vi "LockIn_#1_data.vi"(1 "Choose Lock-In #3":u16(ring) items=["SR830", "PE7265", "LIA7230", "zurichInst"]) -> (0 "String":string)   [LabVIEW 2019]
uses:
  Instrument_Setup.vi
  Global Variables/Data_Display_global.vi
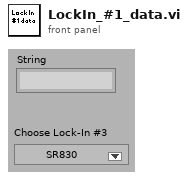
[diagram p1: front panel]
types:
  T1 = typedef "SR830-Settings-Cluster.ctl" = cluster{"VISA":refnum<visa-resource-name>, "Display Channel 2":cluster{" display":i32, " ratio":u16, "output":u16}, "Display Channel 1":cluster{" display":i32, " ratio":u16, "output":u16}, "Time constant":cluster{"time constant\n(10 µs : 0) ":i32, "slope (6 dB/oct)":i32}, "Sensitivity":cluster{"sensitivity\n2nV/fA":i32, "dyn reserve\n(low noise:2)":i16, "ref. phase":ext, "automeasure":bool}, "Offset - Expand.":cluster{"Expand (0: x1)":u16, "Offset/Expand Parameter (1: X)":u16, "Manual Offset (0)":dbl}, "Reference":cluster{"ref. source":bool, "osc.harm# ":u16, "osc. freq":ext, "osc. ampl.":ext, "ref. trigger":u16}, "Lock In 1 sync":cluster{"sync filter":bool, "line filter\n(off:0)":i32}, "Lock In 1 input":cluster{"input":u16, "ground":bool, "couple":bool}}
  T2 = typedef "SR830-Cluster.ctl" = cluster{"Lockin 1":dbl[][], "X1-Display":dbl, "Y1-Display":dbl, "X1 Percent":dbl, "X1 Overload":bool, "Y1 Overload":bool, "Unit X1":string, "Unit X2":string, "Unit X2a":string, "Unit X1a":string, "Sensitivity Setpoint":i16, "X1 Percent 2":dbl, "Y1":dbl, "X1":dbl, "Preamp OVL":bool}
  T3 = typedef "PE7265-Cluster.ctl" = cluster{"Lockin 1":dbl[][], "X1-Display":dbl, "X1 Percent":dbl, "Y1-Display":dbl, "X1 Percent 2":dbl, "Unit X1":string, "Unit X1a":string, "Unit X2":string, "Unit X2a":string, "X1 Overload":bool, "Y1 Overload":bool, "Sensitivity Setpoint":i16, "X1":dbl, "Y1":dbl}
  T4 = cluster{"PE7265 AutoSens at ech step":bool, "PE7265 Sens":i32, "Coupling":bool, "AC Gain":u16, "Auto AC Gain":bool, "Input Device (Voltage Mode)":bool, "Line Frequency":bool, "Input Connector Shells":bool, "PE7265 Input Mode":u16, "Line Frequency\nRejection Filter":u8, "Port":u16, "7265 GPIB Address":i8, "Interface":bool, "Exit":bool, "GPIB Parameter 7260":cluster{"address":string, "delay time":dbl, "mode":i32}, "PE7265 delay after AS":dbl, "VISA session PE7265":refnum<visa-resource-name>, "Slope":u8, "Synchronous TC":bool, "Time Constant":u16, "Reference I/P":u8, "Reference\nHarmonic":u16, "Oscillator Amplitude (Volts rms)":dbl, "Oscillator Frequency (Hz)":dbl, "Ref Unlocked":bool, "Virtual Reference\nMode":bool}
  T5 = typedef "LIA7230-cluster.ctl" = cluster{"Lockin 1":dbl[][], "X1-Display":dbl, "X1 Percent":dbl, "Y1-Display":dbl, "X1 Percent 2":dbl, "Unit X1":string, "Unit X2":string, "X1 Overload":bool, "Y1 Overload":bool, "Sensitivity Setpoint":i16, "X1":dbl, "Y1":dbl, "Channel 3":dbl, "Channel 4":dbl, "Channel 4 Percent":dbl, "Channel 3 Percent ":dbl, "Unit Channel 3":string, "Unit Channel 4":string, "Overload channel 3":bool, "Overload channel 4":bool, "Offsets (ON)":bool, "Sensitivity Setpoint 2":i16}
  T6 = cluster{"Interface":u16, "Port":u16, "Serial Number":string, "IP Address":string, "Line Frequency\nRejection Filter":u8, "Input Mode":u16, "Input Conn. Shells":bool, "Line Frequency":bool, "Auto AC Gain":bool, "AC Gain":u16, "Input Device":bool, "Range":u8, " Auto Sensitivity ":bool, "Auto Measure":bool, "Range 2":u8, " Auto Sensitivity  2":bool, "Slope":u8, "Synchronous TC":bool, "Time Constant":u16, "Slope 2":u8, "Time Constant 2":u16, "Oscillator Amp (V rms)":dbl, "Oscillator Freq (Hz)":dbl, "Reference I/P":u8, "Ref Harm 1":u16, "Ref Harm2":u16, "Virtual Ref.\nMode":bool, "Dual Harmonic/Reference Mode":bool, "Reference Mode":bool, "TRIG OUT\n= Ref Mon":bool, " Auto Phase ":bool, "Reference Phase 1":dbl, "+90 degrees 1":bool, " Auto Phase 2 ":bool, "Reference 2 Phase":dbl, "+90 degrees2":bool, "Auxiliary I/O":bool, "Configuration":bool, "Curve Buffer":bool, "Offsets":bool, "X Channel Offset (%)":sgl, "X Channel Offset":bool, "Y Channel Offset (%)":dbl, "Y Channel Offset":bool, " Auto Offset":bool, "X Channel Offset (%) 2":sgl, "X Channel Offset 2":bool, "Y Channel Offset (%) 2":dbl, "Y Channel Offset 2":bool, " Auto Offset 2":bool, "Display Type channel 1":u16, "Display Type channel 2":u16, "Display Type channel 3":u16, "Display Type channel 4":u16, "Osc Sweeps":bool, "Define Equation1":bool, "Coupling":bool}
  T7 = typedef "Control 3.ctl" = cluster{"Adress":string, "Load Settings from File":bool, "Output_Demod1":enum16{"Aux 1", "Aux 2", "Aux 3", "Aux 4"}, "Input_Demod1":enum16{"Sig In 1", "Curr In 1", "Trigger 1", "Trigger 2", "Aux Out 1", "Aux Out 2", "Aux Out 3", "Aux Out 4", "Aux In 1", "Aux In 2", "Constant"}, "Input_Mode_Demod1":enum16{"single ended", "differential"}, "Bandwith_Mode_Demod1":enum16{"TC", "BW NEP", "BW 3dB"}, "Bandw_Value_demod1":dbl, "Demod1_Range":dbl, "Demod1_Harmonic":dbl, "Trigger_Demod1":enum16{"Manual", "External"}, "osc1_freq":dbl, "osc1_amp":dbl, "Demod1_scaling":dbl, "osc2_freq":dbl, "osc2_amp":dbl, "osc3_freq":dbl, "osc3_amp":dbl, "osc4_freq":dbl, "osc4_amp":dbl, "Demod1_Phase (deg)":dbl, "Demod1_order":ext, "Demod1_coupling":enum16{"DC", "AC"}, "Demod1_shields":enum16{"Ground", "Float"}, "Demod1_input_resistance":enum16{"10M", "50"}, "Demod1_Ref_oscillator":ext, "Demod1_output_imp":enum16{"Disable", "Enable"}, "Demod1_output_diff":enum16{"Disable", "Enable"}, "Demod1_rate":dbl, "Demod1_Output_range":dbl, "Output_Demod2":enum16{"Aux 1", "Aux 2", "Aux 3", "Aux 4"}, "Demod2_input":enum16{"Sig In 1", "Curr In 1", "Trigger 1", "Trigger 2", "Aux Out 1", "Aux Out 2", "Aux Out 3", "Aux Out 4", "Aux In 1", "Aux In 2", "Constant"}, "Input_Mode_Demod2":enum16{"single ended", "differential"}, "Bandwith_Mode_Demod2":enum16{"TC", "BW NEP", "BW 3dB"}, "Bandw_Value_demod2":dbl, "Demod2_Range":dbl, "Demod2_Harmonic":dbl, "Trigger_Demod2":enum16{"Manual", "External"}, "Demod2_scaling":dbl, "Demod2_Phase (deg)":dbl, "Demod2_order":ext, "Demod2_coupling":enum16{"DC", "AC"}, "Demod2_shields":enum16{"Ground", "Float"}, "Demod2_input_resistance":enum16{"10M", "50"}, "Demod2_Ref_oscillator":ext, "Demod2_output_imp":enum16{"Disable", "Enable"}, "Demod2_output_diff":enum16{"Disable", "Enable"}, "Demod2_rate":dbl, "Demod2_Output_range":dbl, "Output_Demod3":enum16{"Aux 1", "Aux 2", "Aux 3", "Aux 4"}, "Demod3_input":enum16{"Sig In 1", "Curr In 1", "Trigger 1", "Trigger 2", "Aux Out 1", "Aux Out 2", "Aux Out 3", "Aux Out 4", "Aux In 1", "Aux In 2", "Constant"}, "Input_Mode_Demod3":enum16{"single ended", "differential"}, "Bandwith_Mode_Demod2":enum16{"TC", "BW NEP", "BW 3dB"}, "Bandw_Value_demod3":dbl, "Demod3_Range":dbl, "Demod3_Harmonic":dbl, "Trigger_Demod3":enum16{"Manual", "External"}, "Demod3_scaling":dbl, "Demod3_Phase (deg)":dbl, "Demod3_order":ext, "Demod3_coupling":enum16{"DC", "AC"}, "Demod3_shields":enum16{"Ground", "Float"}, "Demod3_input_resistance":enum16{"10M", "50"}, "Demod3_Ref_oscillator":ext, "Demod3_output_imp":enum16{"Disable", "Enable"}, "Demod3_output_diff":enum16{"Disable", "Enable"}, "Demod3_rate":dbl, "Demod3_Output_range":dbl, "Output_Demod4":enum16{"Aux 1", "Aux 2", "Aux 3", "Aux 4"}, "Demod4_input":enum16{"Sig In 1", "Curr In 1", "Trigger 1", "Trigger 2", "Aux Out 1", "Aux Out 2", "Aux Out 3", "Aux Out 4", "Aux In 1", "Aux In 2", "Constant"}, "Input_Mode_Demod4":enum16{"single ended", "differential"}, "Bandwith_Mode_Demod4":enum16{"TC", "BW NEP", "BW 3dB"}, "Bandw_Value_demod4":dbl, "Demod4_Range":dbl, "Demod4_Harmonic":dbl, "Trigger_Demod4":enum16{"Manual", "External"}, "Demod4_scaling":dbl, "Demod4_Phase (deg)":dbl, "Demod4_order":ext, "Demod4_coupling":enum16{"DC", "AC"}, "Demod4_shields":enum16{"Ground", "Float"}, "Demod4_input_resistance":enum16{"10M", "50"}, "Demod4_Ref_oscillator":ext, "Demod4_output_imp":enum16{"Disable", "Enable"}, "Demod4_output_diff":enum16{"Disable", "Enable"}, "Demod4_rate":dbl, "Demod4_Output_range":dbl, "Oscillator1_Amp_units":enum16{"Vpk", "Vrms", "VdBm"}, "Oscillator4_Amp_units":enum16{"Vpk", "Vrms", "VdBm"}, "Oscillator2_Amp_units":enum16{"Vpk", "Vrms", "VdBm"}, "Oscillator3_Amp_units":enum16{"Vpk", "Vrms", "VdBm"}, "Demod1_sync_filter":enum16{"Disable", "Enable"}, "Demod 1 (on/off)":bool, "Demod 2 (on/off) ":bool, "Demod 3 (on/off) ":bool, "Demod 4 (on/off) ":bool, " Sigouts 1 (on/off)":bool, " Sigouts 2 (on/off) ":bool, " Sigouts 3 (on/off)":bool, " Sigouts 4 (on/off) ":bool, "Demod2_sync_filter":enum16{"Disable", "Enable"}, "Demod1_auto_outp_rang":enum16{"Disable", "Enable"}, "Demod2_auto_outp_rang ":enum16{"Disable", "Enable"}}
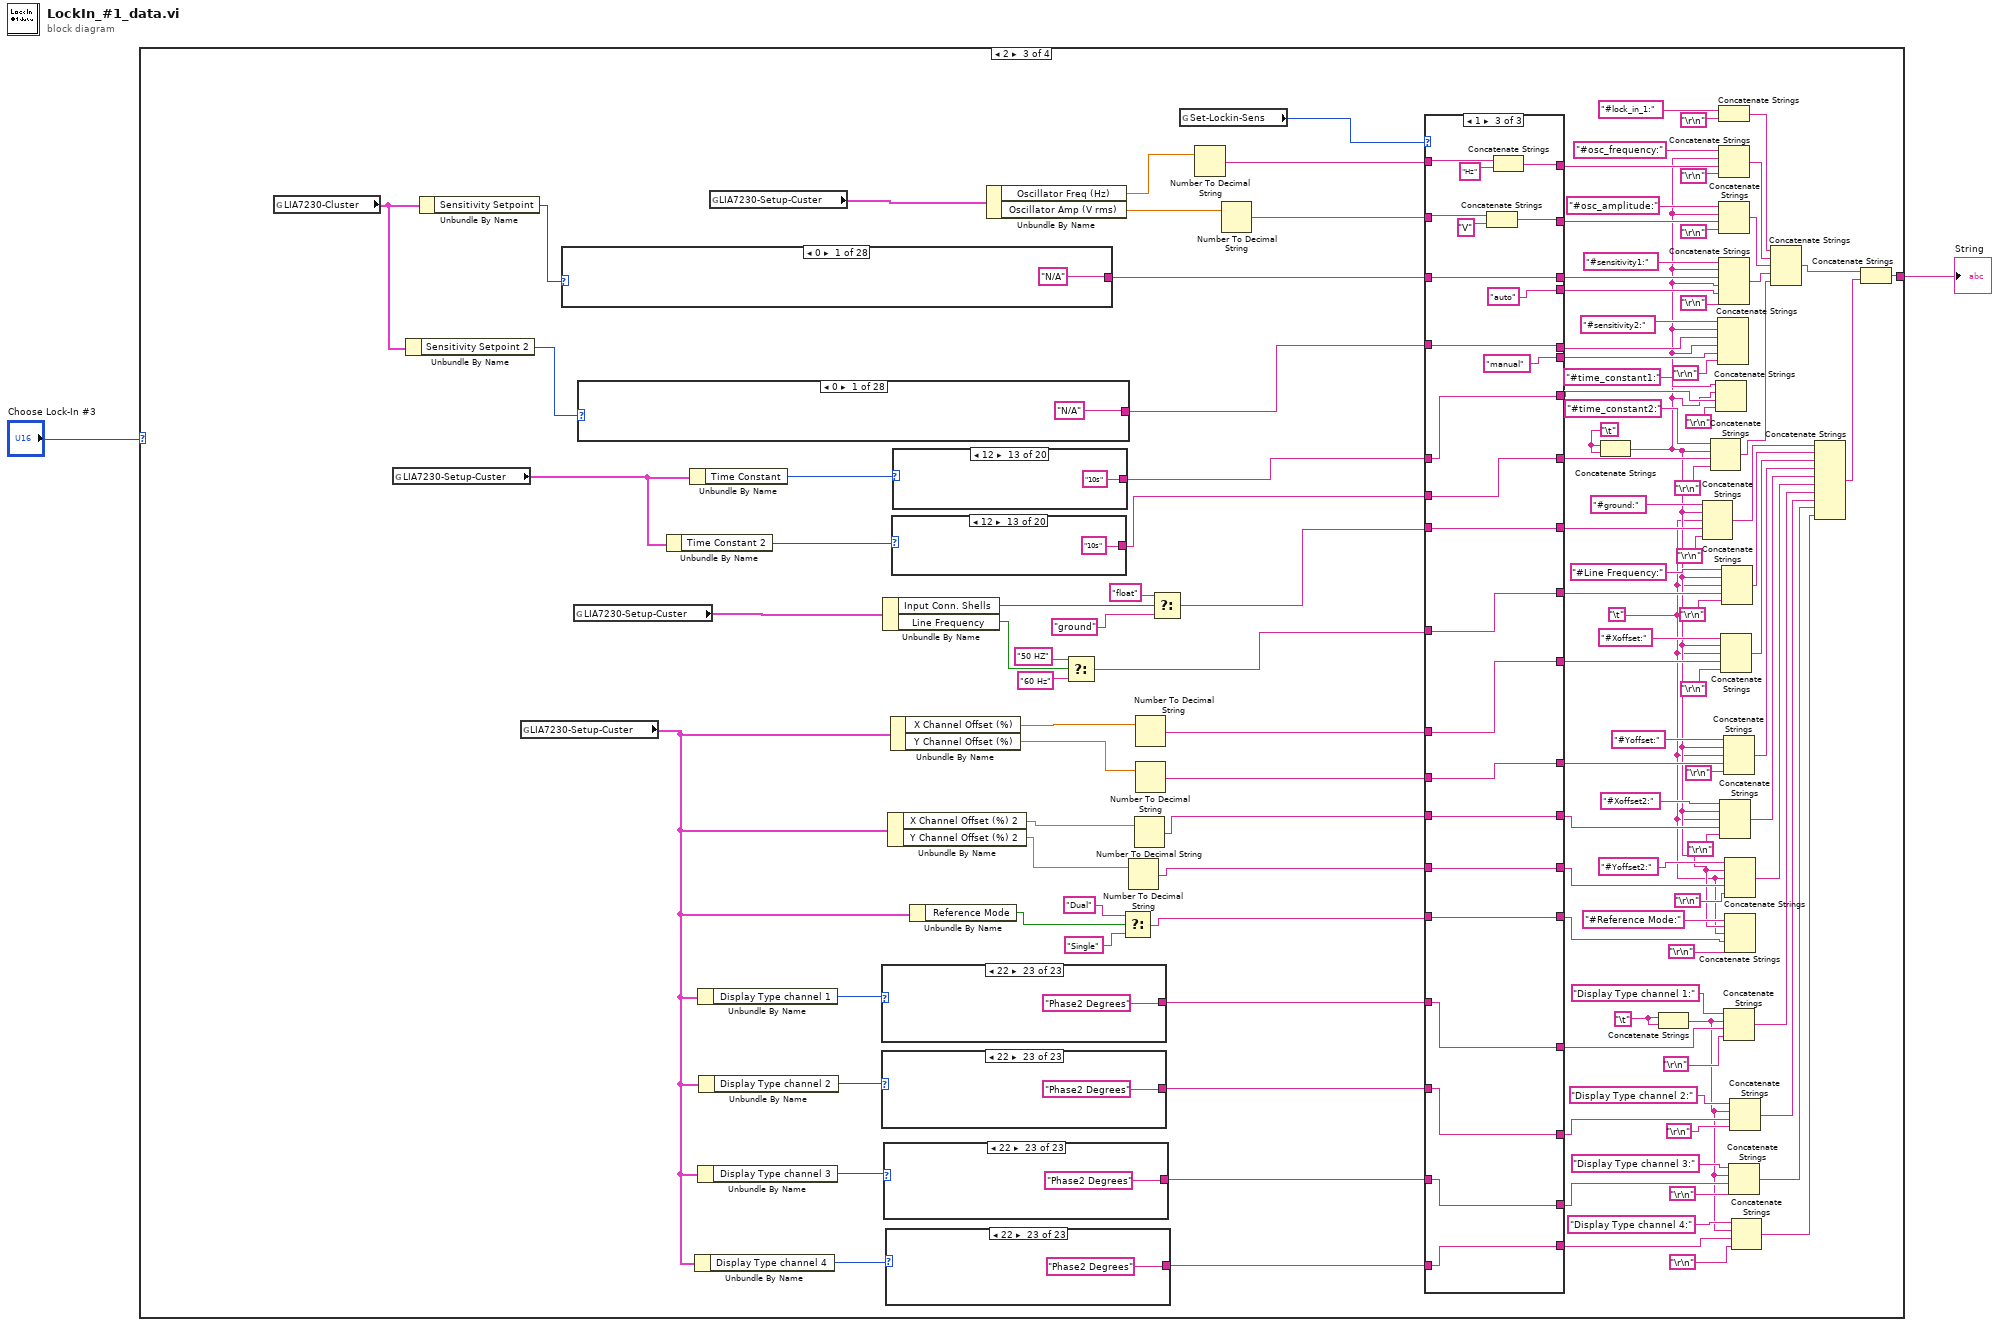
[diagram p0: block diagram]
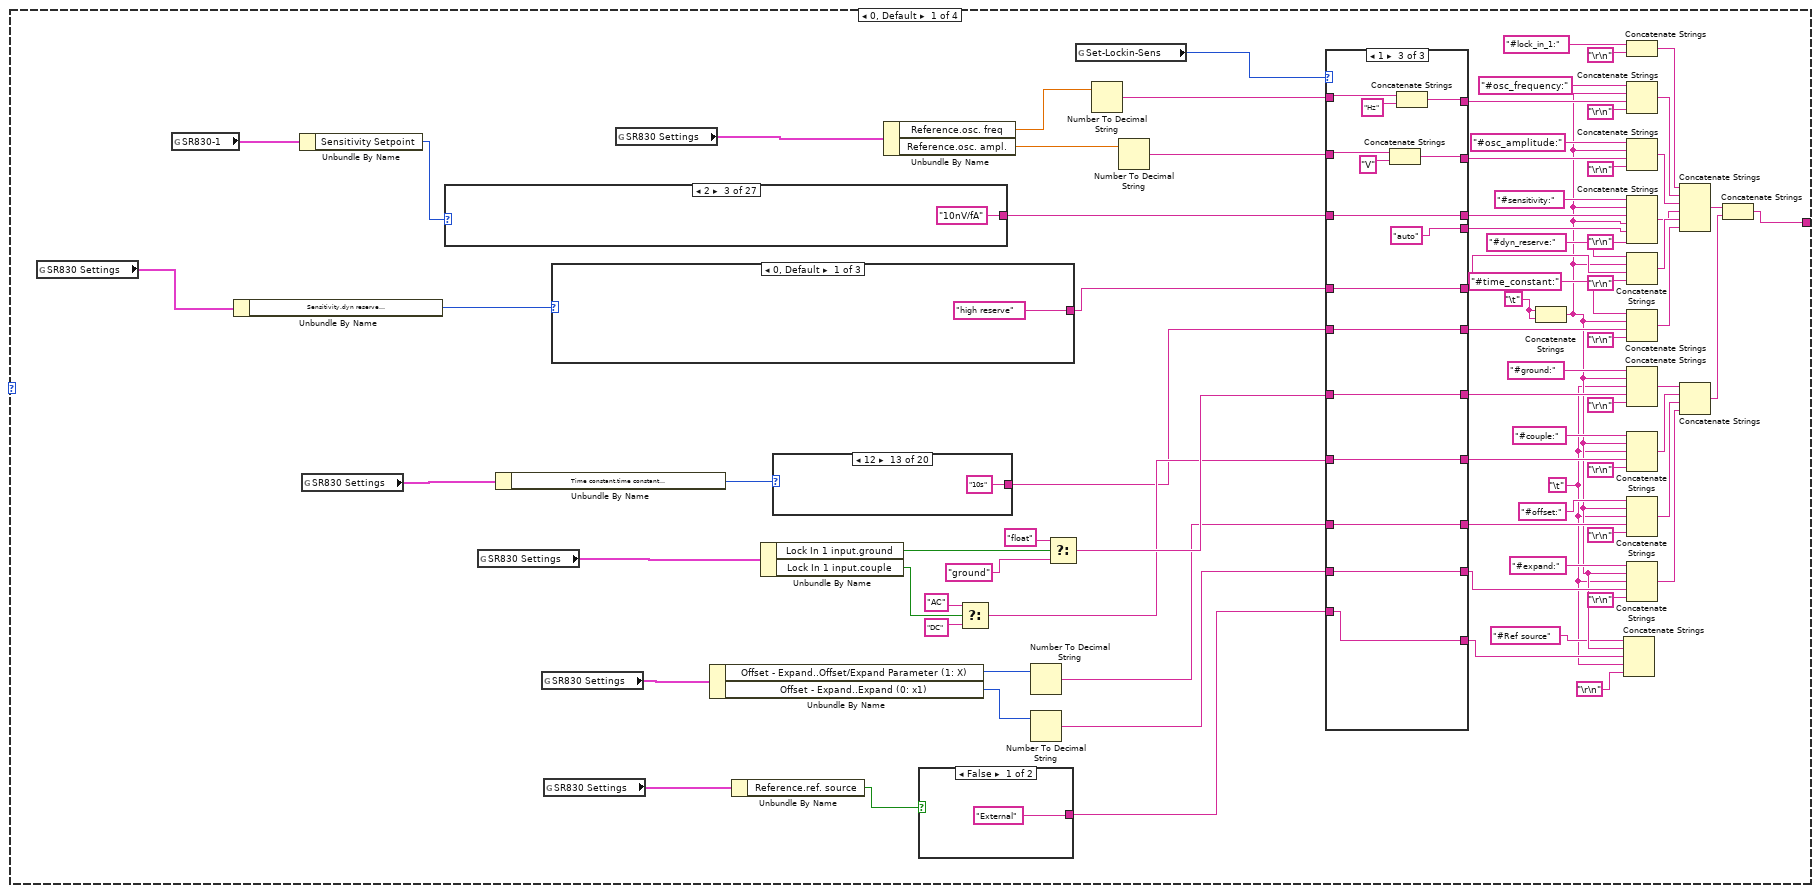
[diagram p2: hidden frame]
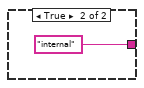
[diagram p3: hidden frame]
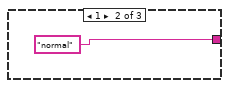
[diagram p4: hidden frame]
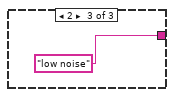
[diagram p5: hidden frame]
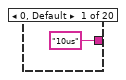
[diagram p6: hidden frame]
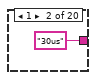
[diagram p7: hidden frame]
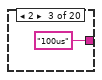
[diagram p8: hidden frame]
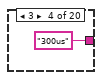
[diagram p9: hidden frame]
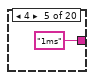
[diagram p10: hidden frame]
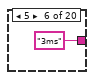
[diagram p11: hidden frame]
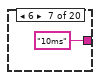
[diagram p12: hidden frame]
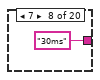
[diagram p13: hidden frame]
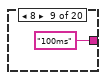
[diagram p14: hidden frame]
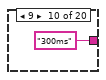
[diagram p15: hidden frame]
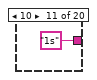
[diagram p16: hidden frame]
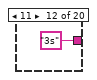
[diagram p17: hidden frame]
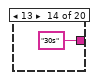
[diagram p18: hidden frame]
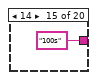
[diagram p19: hidden frame]
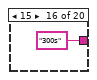
[diagram p20: hidden frame]
diagram:
  n1 = case shown="2" "Choose Lock-In #3" {
    tunnel: [w11 w241 w408 w753] -> w2
    frame 0, Default {
      w3 = "\t"
      w83 = "\t"
      n2 = global read "Instrument_Setup.vi" "SR830 Settings"() -> (w49:T1)
      n3 = global read "Data_Display_global.vi" "SR830-1"() -> (w14:T2)
      n4 = Unbundle By Name(w49) -> ("Sensitivity.dyn reserve\n(low noise:2)"=w16:i16)
      n5 = Unbundle By Name(w14) -> ("Sensitivity Setpoint"=w13:i16)
      n6 = global read "Instrument_Setup.vi" "SR830 Settings"() -> (w55:T1)
      n7 = case shown="2" w13 {
        tunnel: ["2nV/fA" "5nV/fA" "10nV/fA" "20nV/fA" "50nV/fA" "100nV/fA" "200nV/fA" "500nV/fA" "1uV/pA" "2uV/pA" "5uV/pA" "10uV/pA" "20uV/pA" "50uV/pA" "100uV/pA" "200uV/pA" "500uV/pA" "1mV/nA" "2mV/nA" "5mV/nA" "10mV/nA" "20mV/nA" "50mV/nA" "100mV/nA" "200mV/nA" "500mV/nA" "1V/uA"] -> w20
        frame 0, Default {
        }
        frame 1 {
        }
        frame 2 {
        }
        frame 3 {
        }
        frame 4 {
        }
        frame 5 {
        }
        frame 6 {
        }
        frame 7 {
        }
        frame 8 {
        }
        frame 9 {
        }
        frame 10 {
        }
        frame 11 {
        }
        frame 12 {
        }
        frame 13 {
        }
        frame 14 {
        }
        frame 15 {
        }
        frame 16 {
        }
        frame 17 {
        }
        frame 18 {
        }
        frame 19 {
        }
        frame 20 {
        }
        frame 21 {
        }
        frame 22 {
        }
        frame 23 {
        }
        frame 24 {
        }
        frame 25 {
        }
        frame 26 {
        }
      }
      n8 = global read "Instrument_Setup.vi" "SR830 Settings"() -> (w61:T1)
      n9 = Unbundle By Name(w55) -> ("Time constant.time constant\n(10 µs : 0)"=w19:i32)
      n10 = global read "Instrument_Setup.vi" "SR830 Settings"() -> (w68:T1)
      n11 = global read "Instrument_Setup.vi" "SR830 Settings"() -> (w10:T1)
      n12 = case shown="0, Default" w16 {
        tunnel: ["high reserve" "normal" "low noise"] -> w17
        frame 0, Default {
        }
        frame 1 {
        }
        frame 2 {
        }
      }
      n13 = global read "Instrument_Setup.vi" "SR830 Settings"() -> (w47:T1)
      n14 = Unbundle By Name(w68) -> ("Offset - Expand..Offset/Expand Parameter (1: X)"=w40:u16, "Offset - Expand..Expand (0: x1)"=w39:u16)
      n15 = Unbundle By Name(w10) -> ("Reference.ref. source"=w9:bool)
      n16 = Unbundle By Name(w61) -> ("Lock In 1 input.ground"=w62:bool, "Lock In 1 input.couple"=w37:bool)
      n17 = case shown="12" w19 {
        tunnel: ["10us" "30us" "100us" "300us" "1ms" "3ms" "10ms" "30ms" "100ms" "300ms" "1s" "3s" "10s" "30s" "100s" "300s" "1ks" "3ks" "10ks" "30ks"] -> w18
        frame 0, Default {
        }
        frame 1 {
        }
        frame 2 {
        }
        frame 3 {
        }
        frame 4 {
        }
        frame 5 {
        }
        frame 6 {
        }
        frame 7 {
        }
        frame 8 {
        }
        frame 9 {
        }
        frame 10 {
        }
        frame 11 {
        }
        frame 12 {
        }
        frame 13 {
        }
        frame 14 {
        }
        frame 15 {
        }
        frame 16 {
        }
        frame 17 {
        }
        frame 18 {
        }
        frame 19 {
        }
      }
      n18 = Unbundle By Name(w47) -> ("Reference.osc. freq"=w42:ext, "Reference.osc. ampl."=w41:ext)
      n19 = case shown="False" w9 {
        tunnel: ["External" "internal"] -> w8
        frame False {
        }
        frame True {
        }
      }
      n20 = Select(t="AC", s=w37, f="DC") -> (s? t:f=w32:string)
      n21 = Number To Decimal String(number=w40) -> (decimal integer string=w30:string)  [unwired: 1 in]
      n22 = Number To Decimal String(number=w39) -> (decimal integer string=w28:string)  [unwired: 1 in]
      n23 = Select(t="float", s=w62, f="ground") -> (s? t:f=w34:string)
      n24 = global read "Instrument_Setup.vi" "Set-Lockin-Sens"() -> (w36:u16)
      n25 = Number To Decimal String(number=w42) -> (decimal integer string=w26:string)  [unwired: 1 in]
      n26 = Number To Decimal String(number=w41) -> (decimal integer string=w24:string)  [unwired: 1 in]
      n27 = case shown="1" w36 {
        tunnel: w18 -> [w138 w159 w174]
        tunnel: [w138 w159 w174] -> w35
        tunnel: w34 -> [w150 w165 w180]
        tunnel: [w150 w165 w180] -> w33
        tunnel: w32 -> [w149 w164 w179]
        tunnel: [w149 w164 w179] -> w31
        tunnel: [w147 w162 w177] -> w29
        tunnel: w30 -> [w147 w162 w177]
        tunnel: w28 -> [w148 w163 w178]
        tunnel: [w148 w163 w178] -> w27
        tunnel: w26 -> [w145 w155 w170]
        tunnel: [w144 w153 w168] -> w25
        tunnel: w24 -> [w142 w154 w169]
        tunnel: [w141 w152 w167] -> w23
        tunnel: w20 -> [w140 w161 w176]
        tunnel: [w140 w161 w176] -> w22
        tunnel: w17 -> [w139 w160 w175]
        tunnel: [w139 w160 w175] -> w21
        tunnel: ["Command-file" "manual" "auto"] -> w12
        tunnel: w8 -> [w136 w151 w166]
        tunnel: [w136 w151 w166] -> w4
        frame 0, Default {
          n28 = Concatenate Strings(w142, "V" ("String")) -> (w141:string)
          n29 = Concatenate Strings(w145, "Hz" ("String")) -> (w144:string)
        }
        frame 2 {
          n30 = Concatenate Strings(w154, "V" ("String")) -> (w152:string)
          n31 = Concatenate Strings(w155, "Hz" ("String")) -> (w153:string)
        }
        frame 1 {
          n32 = Concatenate Strings(w169, "V" ("String")) -> (w167:string)
          n33 = Concatenate Strings(w170, "Hz" ("String")) -> (w168:string)
        }
      }
      n34 = Concatenate Strings(w83, w83) -> (w6:string)
      n35 = Concatenate Strings("#Ref source", w6, w4, w3, "\r\n") -> ()  [unwired: 1 out]
      n36 = Concatenate Strings("#lock_in_1:", "\r\n") -> (w46:string)
      n37 = Concatenate Strings("#osc_frequency:", w6, w25, "\r\n") -> (w72:string)
      n38 = Concatenate Strings("#osc_amplitude:" ("String"), w6, w23, "\r\n") -> (w73:string)
      n39 = Concatenate Strings("#sensitivity:" ("String"), w6, w22, w6, w12, "\r\n") -> (w74:string)
      n40 = Concatenate Strings("#dyn_reserve:" ("String"), w6, w21, "\r\n") -> (w75:string)
      n41 = Concatenate Strings("#time_constant:" ("String"), w6, w35, "\r\n") -> (w76:string)
      n42 = Concatenate Strings("#ground:" ("String"), w6, w3, w33, "\r\n") -> (w77:string)
      n43 = Concatenate Strings("#couple:" ("String"), w6, w3, w31, "\r\n") -> (w78:string)
      n44 = Concatenate Strings("#offset:" ("String"), w6, w3, w29, "\r\n") -> (w79:string)
      n45 = Concatenate Strings("#expand:" ("String"), w6, w3, w27, "\r\n") -> (w80:string)
      n46 = Concatenate Strings(w46, w72, w73, w74, w75, w76) -> (w81:string)
      n47 = Concatenate Strings(w77, w78, w79, w80) -> (w82:string)
      n48 = Concatenate Strings(w81, w82) -> (w11:string)
    }
    frame 1 {
      w208 = "\t"
      w242 = "\t"
      n49 = global read "Data_Display_global.vi" "PE7265-Cluster"() -> (w187:T3)
      n50 = Unbundle By Name(w187) -> ("Sensitivity Setpoint"=w186:i16)
      n51 = global read "Instrument_Setup.vi" "PE7625-Settings"() -> (w217:T4)
      n52 = case shown="2" w186 {
        tunnel: ["2nV/fA" "5nV/fA" "10nV/fA" "20nV/fA" "50nV/fA" "100nV/fA" "200nV/fA" "500nV/fA" "1uV/pA" "2uV/pA" "5uV/pA" "10uV/pA" "20uV/pA" "50uV/pA" "100uV/pA" "200uV/pA" "500uV/pA" "1mV/nA" "2mV/nA" "5mV/nA" "10mV/nA" "20mV/nA" "50mV/nA" "100mV/nA" "200mV/nA" "500mV/nA" "1V/uA"] -> w191
        frame 0, Default {
        }
        frame 1 {
        }
        frame 2 {
        }
        frame 3 {
        }
        frame 4 {
        }
        frame 5 {
        }
        frame 6 {
        }
        frame 7 {
        }
        frame 8 {
        }
        frame 9 {
        }
        frame 10 {
        }
        frame 11 {
        }
        frame 12 {
        }
        frame 13 {
        }
        frame 14 {
        }
        frame 15 {
        }
        frame 16 {
        }
        frame 17 {
        }
        frame 18 {
        }
        frame 19 {
        }
        frame 20 {
        }
        frame 21 {
        }
        frame 22 {
        }
        frame 23 {
        }
        frame 24 {
        }
        frame 25 {
        }
        frame 26 {
        }
      }
      n53 = global read "Instrument_Setup.vi" "PE7625-Settings"() -> (w223:T4)
      n54 = global read "Instrument_Setup.vi" "PE7625-Settings"() -> (w230:T4)
      n55 = Unbundle By Name(w217) -> ("Time Constant"=w190:u16)
      n56 = global read "Instrument_Setup.vi" "PE7625-Settings"() -> (w212:T4)
      n57 = Unbundle By Name(w230) -> ("AC Gain"=w182:u16)
      n58 = Unbundle By Name(w223) -> ("Input Connector Shells"=w224:bool, "Coupling"=w204:bool)
      n59 = case shown="0, Default" w190 {
        tunnel: ["10us" "20us" "40us" "80us" "160us" "320us" "640us" "5ms" "10ms" "20ms" "50ms" "100ms" "200ms" "500ms" "1s" "2s" "5s" "10s" "20s" "50s" "100s" "200s" "500s" "1ks" "2ks" "5ks" "10ks" "20ks" "50ks" "100ks"] -> w189
        frame 0, Default {
        }
        frame 1 {
        }
        frame 2 {
        }
        frame 3 {
        }
        frame 4 {
        }
        frame 5 {
        }
        frame 6 {
        }
        frame 7 {
        }
        frame 8 {
        }
        frame 9 {
        }
        frame 10 {
        }
        frame 11 {
        }
        frame 12 {
        }
        frame 13 {
        }
        frame 14 {
        }
        frame 15 {
        }
        frame 16 {
        }
        frame 17 {
        }
        frame 18 {
        }
        frame 19 {
        }
        frame 20 {
        }
        frame 21 {
        }
        frame 22 {
        }
        frame 23 {
        }
        frame 24 {
        }
        frame 25 {
        }
        frame 26 {
        }
        frame 27 {
        }
        frame 28 {
        }
        frame 29 {
        }
      }
      n60 = Unbundle By Name(w212) -> ("Oscillator Frequency (Hz)"=w207:dbl, "Oscillator Amplitude (Volts rms)"=w206:dbl)
      n61 = case shown="9" w182 {
        tunnel: ["0dB" "10dB" "20dB" "30dB" "40dB" "50dB" "60dB" "70dB" "80dB" "90dB"] -> w181
        frame 0, Default {
        }
        frame 1 {
        }
        frame 2 {
        }
        frame 3 {
        }
        frame 4 {
        }
        frame 5 {
        }
        frame 6 {
        }
        frame 7 {
        }
        frame 8 {
        }
        frame 9 {
        }
      }
      n62 = Select(t="DC", s=w204, f="AC") -> (s? t:f=w199:string)
      n63 = Select(t="float", s=w224, f="ground") -> (s? t:f=w201:string)
      n64 = global read "Instrument_Setup.vi" "Set-Lockin-Sens"() -> (w203:u16)
      n65 = Number To Decimal String(number=w207) -> (decimal integer string=w196:string)  [unwired: 1 in]
      n66 = Number To Decimal String(number=w206) -> (decimal integer string=w194:string)  [unwired: 1 in]
      n67 = case shown="1" w203 {
        tunnel: w189 -> [w311 w329 w341]
        tunnel: [w311 w329 w341] -> w202
        tunnel: w201 -> [w321 w333 w345]
        tunnel: [w321 w333 w345] -> w200
        tunnel: w199 -> [w320 w332 w344]
        tunnel: [w320 w332 w344] -> w198
        tunnel: [w319 w331 w343] -> w197
        tunnel: w181 -> [w319 w331 w343]
        tunnel: w196 -> [w317 w325 w337]
        tunnel: [w316 w323 w335] -> w195
        tunnel: w194 -> [w314 w324 w336]
        tunnel: [w313 w322 w334] -> w193
        tunnel: w191 -> [w312 w330 w342]
        tunnel: [w312 w330 w342] -> w192
        tunnel: ["Command-file" "manual" "auto"] -> w184
        frame 0, Default {
          n68 = Concatenate Strings(w314, "V" ("String")) -> (w313:string)
          n69 = Concatenate Strings(w317, "Hz" ("String")) -> (w316:string)
        }
        frame 2 {
          n70 = Concatenate Strings(w324, "V" ("String")) -> (w322:string)
          n71 = Concatenate Strings(w325, "Hz" ("String")) -> (w323:string)
        }
        frame 1 {
          n72 = Concatenate Strings(w336, "V" ("String")) -> (w334:string)
          n73 = Concatenate Strings(w337, "Hz" ("String")) -> (w335:string)
        }
      }
      n74 = Concatenate Strings(w242, w242) -> (w185:string)
      n75 = Concatenate Strings("#lock_in_1:", "\r\n") -> (w211:string)
      n76 = Concatenate Strings("#osc_frequency:", w185, w195, "\r\n") -> (w233:string)
      n77 = Concatenate Strings("#osc_amplitude:" ("String"), w185, w193, "\r\n") -> (w234:string)
      n78 = Concatenate Strings("#sensitivity:" ("String"), w185, w192, w185, w184, "\r\n") -> (w235:string)
      n79 = Concatenate Strings("#time_constant:" ("String"), w185, w202, "\r\n") -> (w183:string)
      n80 = Concatenate Strings("#ground:" ("String"), w185, w208, w200, "\r\n") -> (w236:string)
      n81 = Concatenate Strings("#couple:" ("String"), w185, w208, w198, "\r\n") -> (w237:string)
      n82 = Concatenate Strings("#AC Gain" ("String"), w185, w208, w197, "\r\n") -> (w238:string)
      n83 = Concatenate Strings(w211, w233, w234, w235, w183) -> (w239:string)
      n84 = Concatenate Strings(w236, w237, w238) -> (w240:string)
      n85 = Concatenate Strings(w239, w240) -> (w241:string)
    }
    frame 2 {
      w362 = "\t"
      w374 = "\t"
      w469 = "\t"
      n86 = global read "Data_Display_global.vi" "LIA7230-Cluster"() -> (w407:T5)
      n87 = global read "Instrument_Setup.vi" "LIA7230-Setup-Custer"() -> (w399:T6)
      n88 = Unbundle By Name(w407) -> ("Sensitivity Setpoint 2"=w406:i16)
      n89 = Unbundle By Name(w407) -> ("Sensitivity Setpoint"=w410:i16)
      n90 = global read "Instrument_Setup.vi" "LIA7230-Setup-Custer"() -> (w371:T6)
      n91 = case shown="0" w410 {
        tunnel: ["N/A" "2nV/fA" "5nV/fA" "10nV/fA" "20nV/fA" "50nV/fA" "100nV/fA" "200nV/fA" "500nV/fA" "1uV/pA" "2uV/pA" "5uV/pA" "10uV/pA" "20uV/pA" "50uV/pA" "100uV/pA" "200uV/pA" "500uV/pA" "1mV/nA" "2mV/nA" "5mV/nA" "10mV/nA" "20mV/nA" "50mV/nA" "100mV/nA" "200mV/nA" "500mV/nA" "1V/uA"] -> w414
        frame 0 {
        }
        frame 1, Default {
        }
        frame 2 {
        }
        frame 3 {
        }
        frame 4 {
        }
        frame 5 {
        }
        frame 6 {
        }
        frame 7 {
        }
        frame 8 {
        }
        frame 9 {
        }
        frame 10 {
        }
        frame 11 {
        }
        frame 12 {
        }
        frame 13 {
        }
        frame 14 {
        }
        frame 15 {
        }
        frame 16 {
        }
        frame 17 {
        }
        frame 18 {
        }
        frame 19 {
        }
        frame 20 {
        }
        frame 21 {
        }
        frame 22 {
        }
        frame 23 {
        }
        frame 24 {
        }
        frame 25 {
        }
        frame 26 {
        }
        frame 27 {
        }
      }
      n92 = global read "Instrument_Setup.vi" "LIA7230-Setup-Custer"() -> (w450:T6)
      n93 = case shown="0" w406 {
        tunnel: ["N/A" "2nV/fA" "5nV/fA" "10nV/fA" "20nV/fA" "50nV/fA" "100nV/fA" "200nV/fA" "500nV/fA" "1uV/pA" "2uV/pA" "5uV/pA" "10uV/pA" "20uV/pA" "50uV/pA" "100uV/pA" "200uV/pA" "500uV/pA" "1mV/nA" "2mV/nA" "5mV/nA" "10mV/nA" "20mV/nA" "50mV/nA" "100mV/nA" "200mV/nA" "500mV/nA" "1V/uA"] -> w405
        frame 0 {
        }
        frame 1, Default {
        }
        frame 2 {
        }
        frame 3 {
        }
        frame 4 {
        }
        frame 5 {
        }
        frame 6 {
        }
        frame 7 {
        }
        frame 8 {
        }
        frame 9 {
        }
        frame 10 {
        }
        frame 11 {
        }
        frame 12 {
        }
        frame 13 {
        }
        frame 14 {
        }
        frame 15 {
        }
        frame 16 {
        }
        frame 17 {
        }
        frame 18 {
        }
        frame 19 {
        }
        frame 20 {
        }
        frame 21 {
        }
        frame 22 {
        }
        frame 23 {
        }
        frame 24 {
        }
        frame 25 {
        }
        frame 26 {
        }
        frame 27 {
        }
      }
      n94 = Unbundle By Name(w399) -> ("Time Constant 2"=w398:u16)
      n95 = Unbundle By Name(w399) -> ("Time Constant"=w413:u16)
      n96 = Unbundle By Name(w371) -> ("Display Type channel 4"=w368:u16)
      n97 = Unbundle By Name(w371) -> ("Display Type channel 1"=w372:u16)
      n98 = Unbundle By Name(w371) -> ("Display Type channel 3"=w369:u16)
      n99 = Unbundle By Name(w371) -> ("Display Type channel 2"=w370:u16)
      n100 = global read "Instrument_Setup.vi" "LIA7230-Setup-Custer"() -> (w440:T6)
      n101 = case shown="22" w372 {
        tunnel: ["X%" "Y%" "X Calibrated" "Y Calibrated" "Mag %" "Mag Calibrated" "Phase Degree" "Ratio" "Log Ratio" "ADC 1" "ADC 2" "ADC 3" "ADC 4" "Noise %" "Noise Calibrated" "Ref Frequency" "Equation 1" "Equation 2" "X2 %" "Y2 %" "Mag2 %" "Mag2 Calibrated" "Phase2 Degrees"] -> w367
        frame 0, Default {
        }
        frame 1 {
        }
        frame 2 {
        }
        frame 3 {
        }
        frame 4 {
        }
        frame 5 {
        }
        frame 6 {
        }
        frame 7 {
        }
        frame 8 {
        }
        frame 9 {
        }
        frame 10 {
        }
        frame 11 {
        }
        frame 12 {
        }
        frame 13 {
        }
        frame 14 {
        }
        frame 15 {
        }
        frame 16 {
        }
        frame 17 {
        }
        frame 18 {
        }
        frame 19 {
        }
        frame 20 {
        }
        frame 21 {
        }
        frame 22 {
        }
      }
      n102 = case shown="22" w370 {
        tunnel: ["X%" "Y%" "X Calibrated" "Y Calibrated" "Mag %" "Mag Calibrated" "Phase Degree" "Ratio" "Log Ratio" "ADC 1" "ADC 2" "ADC 3" "ADC 4" "Noise %" "Noise Calibrated" "Ref Frequency" "Equation 1" "Equation 2" "X2 %" "Y2 %" "Mag2 %" "Mag2 Calibrated" "Phase2 Degrees"] -> w366
        frame 0, Default {
        }
        frame 1 {
        }
        frame 2 {
        }
        frame 3 {
        }
        frame 4 {
        }
        frame 5 {
        }
        frame 6 {
        }
        frame 7 {
        }
        frame 8 {
        }
        frame 9 {
        }
        frame 10 {
        }
        frame 11 {
        }
        frame 12 {
        }
        frame 13 {
        }
        frame 14 {
        }
        frame 15 {
        }
        frame 16 {
        }
        frame 17 {
        }
        frame 18 {
        }
        frame 19 {
        }
        frame 20 {
        }
        frame 21 {
        }
        frame 22 {
        }
      }
      n103 = Unbundle By Name(w450) -> ("Input Conn. Shells"=w451:bool, "Line Frequency"=w430:bool)
      n104 = case shown="22" w369 {
        tunnel: ["X%" "Y%" "X Calibrated" "Y Calibrated" "Mag %" "Mag Calibrated" "Phase Degree" "Ratio" "Log Ratio" "ADC 1" "ADC 2" "ADC 3" "ADC 4" "Noise %" "Noise Calibrated" "Ref Frequency" "Equation 1" "Equation 2" "X2 %" "Y2 %" "Mag2 %" "Mag2 Calibrated" "Phase2 Degrees"] -> w365
        frame 0, Default {
        }
        frame 1 {
        }
        frame 2 {
        }
        frame 3 {
        }
        frame 4 {
        }
        frame 5 {
        }
        frame 6 {
        }
        frame 7 {
        }
        frame 8 {
        }
        frame 9 {
        }
        frame 10 {
        }
        frame 11 {
        }
        frame 12 {
        }
        frame 13 {
        }
        frame 14 {
        }
        frame 15 {
        }
        frame 16 {
        }
        frame 17 {
        }
        frame 18 {
        }
        frame 19 {
        }
        frame 20 {
        }
        frame 21 {
        }
        frame 22 {
        }
      }
      n105 = case shown="22" w368 {
        tunnel: ["X%" "Y%" "X Calibrated" "Y Calibrated" "Mag %" "Mag Calibrated" "Phase Degree" "Ratio" "Log Ratio" "ADC 1" "ADC 2" "ADC 3" "ADC 4" "Noise %" "Noise Calibrated" "Ref Frequency" "Equation 1" "Equation 2" "X2 %" "Y2 %" "Mag2 %" "Mag2 Calibrated" "Phase2 Degrees"] -> w364
        frame 0, Default {
        }
        frame 1 {
        }
        frame 2 {
        }
        frame 3 {
        }
        frame 4 {
        }
        frame 5 {
        }
        frame 6 {
        }
        frame 7 {
        }
        frame 8 {
        }
        frame 9 {
        }
        frame 10 {
        }
        frame 11 {
        }
        frame 12 {
        }
        frame 13 {
        }
        frame 14 {
        }
        frame 15 {
        }
        frame 16 {
        }
        frame 17 {
        }
        frame 18 {
        }
        frame 19 {
        }
        frame 20 {
        }
        frame 21 {
        }
        frame 22 {
        }
      }
      n106 = Unbundle By Name(w371) -> ("X Channel Offset (%) 2"=w391:sgl, "Y Channel Offset (%) 2"=w387:dbl)
      n107 = Unbundle By Name(w371) -> ("X Channel Offset (%)"=w433:sgl, "Y Channel Offset (%)"=w432:dbl)
      n108 = case shown="12" w398 {
        tunnel: ["10us" "30us" "100us" "300us" "1ms" "3ms" "10ms" "30ms" "100ms" "300ms" "1s" "3s" "10s" "30s" "100s" "300s" "1ks" "3ks" "10ks" "30ks"] -> w397
        frame 0, Default {
        }
        frame 1 {
        }
        frame 2 {
        }
        frame 3 {
        }
        frame 4 {
        }
        frame 5 {
        }
        frame 6 {
        }
        frame 7 {
        }
        frame 8 {
        }
        frame 9 {
        }
        frame 10 {
        }
        frame 11 {
        }
        frame 12 {
        }
        frame 13 {
        }
        frame 14 {
        }
        frame 15 {
        }
        frame 16 {
        }
        frame 17 {
        }
        frame 18 {
        }
        frame 19 {
        }
      }
      n109 = case shown="12" w413 {
        tunnel: ["10us" "30us" "100us" "300us" "1ms" "3ms" "10ms" "30ms" "100ms" "300ms" "1s" "3s" "10s" "30s" "100s" "300s" "1ks" "3ks" "10ks" "30ks"] -> w412
        frame 0, Default {
        }
        frame 1 {
        }
        frame 2 {
        }
        frame 3 {
        }
        frame 4 {
        }
        frame 5 {
        }
        frame 6 {
        }
        frame 7 {
        }
        frame 8 {
        }
        frame 9 {
        }
        frame 10 {
        }
        frame 11 {
        }
        frame 12 {
        }
        frame 13 {
        }
        frame 14 {
        }
        frame 15 {
        }
        frame 16 {
        }
        frame 17 {
        }
        frame 18 {
        }
        frame 19 {
        }
      }
      n110 = Unbundle By Name(w371) -> ("Reference Mode"=w381:bool)
      n111 = Unbundle By Name(w440) -> ("Oscillator Freq (Hz)"=w435:dbl, "Oscillator Amp (V rms)"=w434:dbl)
      n112 = Select(t="50 HZ", s=w430, f="60 Hz") -> (s? t:f=w425:string)
      n113 = Select(t="Dual", s=w381, f="Single") -> (s? t:f=w378:string)
      n114 = Number To Decimal String(number=w387) -> (decimal integer string=w386:string)  [unwired: 1 in]
      n115 = Number To Decimal String(number=w391) -> (decimal integer string=w390:string)  [unwired: 1 in]
      n116 = Number To Decimal String(number=w433) -> (decimal integer string=w423:string)  [unwired: 1 in]
      n117 = Number To Decimal String(number=w432) -> (decimal integer string=w421:string)  [unwired: 1 in]
      n118 = Select(t="float", s=w451, f="ground") -> (s? t:f=w427:string)
      n119 = global read "Instrument_Setup.vi" "Set-Lockin-Sens"() -> (w429:u16)
      n120 = Number To Decimal String(number=w435) -> (decimal integer string=w419:string)  [unwired: 1 in]
      n121 = Number To Decimal String(number=w434) -> (decimal integer string=w417:string)  [unwired: 1 in]
      n122 = case shown="1" w429 {
        tunnel: w412 -> [w666 w689 w712]
        tunnel: [w665 w688 w711] -> w428
        tunnel: w427 -> [w680 w703 w726]
        tunnel: [w680 w703 w726] -> w426
        tunnel: w425 -> [w679 w702 w725]
        tunnel: [w679 w702 w725] -> w424
        tunnel: [w677 w700 w723] -> w422
        tunnel: w423 -> [w677 w700 w723]
        tunnel: w421 -> [w678 w701 w724]
        tunnel: [w678 w701 w724] -> w420
        tunnel: w419 -> [w675 w695 w718]
        tunnel: [w674 w693 w716] -> w418
        tunnel: w417 -> [w672 w694 w717]
        tunnel: [w671 w692 w715] -> w416
        tunnel: w414 -> [w670 w699 w722]
        tunnel: [w670 w699 w722] -> w415
        tunnel: ["Command-file" "manual" "auto"] -> w409
        tunnel: w405 -> [w668 w691 w714]
        tunnel: [w668 w691 w714] -> w402
        tunnel: ["manual" "manual" "manual"] -> w401
        tunnel: w397 -> [w665 w688 w711]
        tunnel: [w666 w689 w712] -> w394
        tunnel: w390 -> [w664 w687 w710]
        tunnel: [w664 w687 w710] -> w389
        tunnel: w386 -> [w663 w686 w709]
        tunnel: [w663 w686 w709] -> w383
        tunnel: w378 -> [w662 w685 w708]
        tunnel: [w662 w685 w708] -> w373
        tunnel: w367 -> [w661 w684 w707]
        tunnel: w366 -> [w660 w683 w706]
        tunnel: w365 -> [w659 w682 w705]
        tunnel: w364 -> [w658 w681 w704]
        tunnel: [w661 w684 w707] -> w361
        tunnel: [w660 w683 w706] -> w358
        tunnel: [w659 w682 w705] -> w355
        tunnel: [w658 w681 w704] -> w351
        frame 0, Default {
          n123 = Concatenate Strings(w672, "V" ("String")) -> (w671:string)
          n124 = Concatenate Strings(w675, "Hz" ("String")) -> (w674:string)
        }
        frame 2 {
          n125 = Concatenate Strings(w694, "V" ("String")) -> (w692:string)
          n126 = Concatenate Strings(w695, "Hz" ("String")) -> (w693:string)
        }
        frame 1 {
          n127 = Concatenate Strings(w717, "V" ("String")) -> (w715:string)
          n128 = Concatenate Strings(w718, "Hz" ("String")) -> (w716:string)
        }
      }
      n129 = Concatenate Strings(w469, w469) -> (w375:string)
      n130 = Concatenate Strings(w362, w362) -> (w352:string)
      n131 = Concatenate Strings("#ground:" ("String"), w375, w374, w426, "\r\n") -> (w463:string)
      n132 = Concatenate Strings("#time_constant2:" ("String"), w375, w428, "\r\n") -> (w400:string)
      n133 = Concatenate Strings("#time_constant1:" ("String"), w375, w394, "\r\n") -> ()  [unwired: 1 out]
      n134 = Concatenate Strings("#sensitivity2:" ("String"), w375, w402, w375, w401, "\r\n") -> ()  [unwired: 1 out]
      n135 = Concatenate Strings("#lock_in_1:", "\r\n") -> (w439:string)
      n136 = Concatenate Strings("#osc_frequency:", w375, w418, "\r\n") -> (w460:string)
      n137 = Concatenate Strings("#osc_amplitude:" ("String"), w375, w416, "\r\n") -> (w461:string)
      n138 = Concatenate Strings("#sensitivity1:" ("String"), w375, w415, w375, w409, "\r\n") -> (w462:string)
      n139 = Concatenate Strings("#Xoffset2:" ("String"), w375, w374, w389, "\r\n") -> (w393:string)
      n140 = Concatenate Strings("#Xoffset:" ("String"), w375, w374, w422, "\r\n") -> (w465:string)
      n141 = Concatenate Strings("#Line Frequency:" ("String"), w375, w374, w424, "\r\n") -> (w464:string)
      n142 = Concatenate Strings("#Yoffset:" ("String"), w375, w374, w420, "\r\n") -> (w466:string)
      n143 = Concatenate Strings("Display Type channel 1:", w352, w361, "\r\n") -> (w349:string)
      n144 = Concatenate Strings("#Yoffset2:" ("String"), w375, w374, w383, "\r\n") -> (w385:string)
      n145 = Concatenate Strings("#Reference Mode:" ("String"), w375, w374, w373, "\r\n") -> ()  [unwired: 1 out]
      n146 = Concatenate Strings("Display Type channel 3:", w352, w355, "\r\n") -> (w347:string)
      n147 = Concatenate Strings("Display Type channel 2:", w352, w358, "\r\n") -> (w348:string)
      n148 = Concatenate Strings("Display Type channel 4:", w352, w351, "\r\n") -> (w346:string)
      n149 = Concatenate Strings(w439, w460, w461, w462, w400) -> (w467:string)
      n150 = Concatenate Strings(w463, w464, w465, w466, w393, w385, w349, w348, w347, w346) -> (w468:string)
      n151 = Concatenate Strings(w467, w468) -> (w408:string)
    }
    frame 3 {
      w763 = "\t"
      w787 = "\t"
      n152 = global read "Instrument_Setup.vi" "zurichInst-1-Settings"() -> (w732:T7)
      n153 = Unbundle By Name(w732) -> ("osc1_freq"=w750:dbl, "osc1_amp"=w748:dbl)
      n154 = Unbundle By Name(w732) -> ("osc2_freq"=w746:dbl, "osc2_amp"=w745:dbl)
      n155 = Unbundle By Name(w732) -> ("Demod1_shields"=w734:enum16{"Ground", "Float"})
      n156 = Unbundle By Name(w732) -> ("Demod1_coupling"=w731:enum16{"DC", "AC"})
      n157 = Number To Decimal String(number=w750) -> (decimal integer string=w749:string)  [unwired: 1 in]
      n158 = Number To Decimal String(number=w748) -> (decimal integer string=w747:string)  [unwired: 1 in]
      n159 = Number To Decimal String(number=w745) -> (decimal integer string=w743:string)  [unwired: 1 in]
      n160 = Number To Decimal String(number=w746) -> (decimal integer string=w744:string)  [unwired: 1 in]
      n161 = case shown="\"Float\"" w734 {
        tunnel: ["Ground" "Float"] -> w733
        frame "Ground", Default {
        }
        frame "Float" {
        }
      }
      n162 = case shown="\"DC\", Default" w731 {
        tunnel: ["DC" "AC"] -> w730
        frame "DC", Default {
        }
        frame "AC" {
        }
      }
      n163 = case shown="2" 1 {
        tunnel: "Not implementet yet" -> [w799 w823 w841]
        tunnel: [w799 w823 w841] -> w762
        tunnel: w733 -> [w809 w827 w845]
        tunnel: [w809 w827 w845] -> w761
        tunnel: w730 -> [w808 w826 w844]
        tunnel: [w808 w826 w844] -> w760
        tunnel: [w807 w825 w843] -> w759
        tunnel: "Not implementet yet" -> [w807 w825 w843]
        tunnel: w749 -> [w805 w819 w837]
        tunnel: [w804 w817 w835] -> w758
        tunnel: w747 -> [w802 w818 w836]
        tunnel: [w801 w816 w834] -> w757
        tunnel: "Nd" -> [w800 w824 w842]
        tunnel: [w800 w824 w842] -> w756
        tunnel: ["Command-file" "manual" "auto"] -> w754
        tunnel: w744 -> [w797 w814 w833]
        tunnel: w743 -> [w796 w813 w831]
        tunnel: [w795 w812 w829] -> w741
        tunnel: [w794 w811 w828] -> w737
        frame 0, Default {
          n164 = Concatenate Strings(w802, "V" ("String")) -> (w801:string)
          n165 = Concatenate Strings(w805, "Hz" ("String")) -> (w804:string)
          n166 = Concatenate Strings(w796, "V" ("String")) -> (w794:string)
          n167 = Concatenate Strings(w797, "Hz" ("String")) -> (w795:string)
        }
        frame 2 {
          n168 = Concatenate Strings(w818, "V" ("String")) -> (w816:string)
          n169 = Concatenate Strings(w813, "V" ("String")) -> (w811:string)
          n170 = Concatenate Strings(w814, "Hz" ("String")) -> (w812:string)
          n171 = Concatenate Strings(w819, "Hz" ("String")) -> (w817:string)
        }
        frame 1 {
          n172 = Concatenate Strings(w837, "Hz" ("String")) -> (w835:string)
          n173 = Concatenate Strings(w831, "V" ("String")) -> (w828:string)
          n174 = Concatenate Strings(w833, "Hz" ("String")) -> (w829:string)
          n175 = Concatenate Strings(w836, "V" ("String")) -> (w834:string)
        }
      }
      n176 = Concatenate Strings(w787, w787) -> (w738:string)
      n177 = Concatenate Strings("#osc2_amplitude:" ("String"), w738, w737, "\r\n") -> ()  [unwired: 1 out]
      n178 = Concatenate Strings("#osc2_frequency:", w738, w741, "\r\n") -> ()  [unwired: 1 out]
      n179 = Concatenate Strings("#time_constant:" ("String"), w738, w762, "\r\n") -> (w727:string)
      n180 = Concatenate Strings("#ground_Demod1:" ("String"), w738, w763, w761, "\r\n") -> (w782:string)
      n181 = Concatenate Strings("#couple_Demod1:" ("String"), w738, w763, w760, "\r\n") -> (w783:string)
      n182 = Concatenate Strings("#AC Gain" ("String"), w738, w763, w759, "\r\n") -> (w784:string)
      n183 = Concatenate Strings("#osc1_amplitude:" ("String"), w738, w757, "\r\n") -> (w781:string)
      n184 = Concatenate Strings("#osc1_frequency:", w738, w758, "\r\n") -> (w780:string)
      n185 = Concatenate Strings("#lock_in_1:", "\r\n") -> (w766:string)
      n186 = Concatenate Strings("#sensitivity:" ("String"), w738, w756, w738, w754, "\r\n") -> (w728:string)
      n187 = Concatenate Strings(w766, w780, w781, w728, w727) -> (w785:string)
      n188 = Concatenate Strings(w782, w783, w784) -> (w786:string)
      n189 = Concatenate Strings(w785, w786) -> (w753:string)
    }
  }
  "String" <- w2
